vi "Configure Modulation Low Level (Frequency).vi"(8 "error in (no error)":errorcluster, 9 "Frequency (100.00 Hz)":dbl=100.0, 10 "Modulation (AM)":enum16{"AM", "FM", "PM", "FSK", "PWM"}(ring), 11 "VISA resource name":refnum<visa-resource-name>) -> (0 "error out":errorcluster, 3 "VISA resource name out":refnum<visa-resource-name>)   [LabVIEW 2017, in "Keithley 3390.lvlib"]
uses:
  Keithley 3390.lvlib
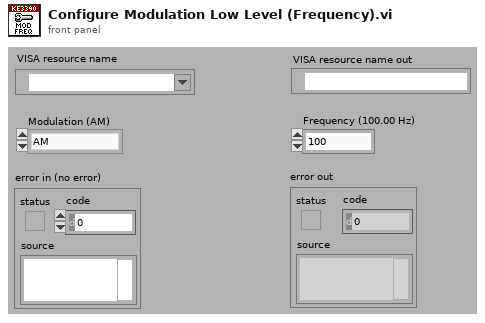
[diagram p1: front panel]
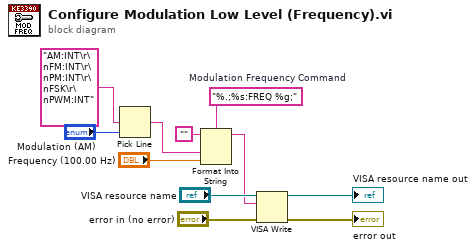
[diagram p0: block diagram]
diagram:
  w7 = "%.;%s:FREQ %g;"  # Modulation Frequency Command
  n1 = Pick Line(multi-line string="AM:INT\r\nFM:INT\r\nPM:INT\r\nFSK\r\nPWM:INT" ("options"), line index="Modulation (AM)") -> (output string=w6:string)  [unwired: 1 in]
  n2 = Format Into String(format string=w7, initial string="", w6, "Frequency (100.00 Hz)") -> (resulting string=w3:string)  [unwired: 1 in, 1 out]
  n3 = VISA Write(VISA resource name="VISA resource name", write buffer=w3, error in (no error)="error in (no error)") -> (VISA resource name out=→"VISA resource name out":refnum<visa-resource-name>, error out=→"error out":errorcluster)  [unwired: 1 out]
